vi "1. Basic retrieve Rulers.vi"() -> ()   [LabVIEW 2017]
uses:
  40fc1cc9-77e3-4a14-9bb9-de70462c7f35.vi
  81b41104-5ca5-45e9-a143-87b761583821.vi
  83982d16-e29d-493a-892c-93b6b063dd3a.vi
  d59d594f-6358-4fe9-a0ea-ade5f599e91a.vi
  177f037c-d6c1-4684-97ba-f775e359171c.vi
  f8914412-5770-4d7c-8ed9-34d3b6c64140.vi
  0842be61-58c2-4c06-9355-20aaf40be817.vi
  a49a9376-e1ff-4fda-bff8-7fdb6b491f6f.vi
  efc68658-e21b-4998-9bfe-a9de0054dd82.vi
  38ed8c4c-bfe5-4ceb-af5c-8de10cee5e52.vi
  a345cc07-d10f-4275-8a18-17707c3f89e9.vi
  cabc4c38-4671-4b03-9489-31c074b0dc0c.vi
  API-String-Arugments-Support/_Support/Convert API String Arguments to Data(variant).vi
panel:
  out "output cluster 11":T1={"API String"="[3.12,4.113,2.3,5;3.12,5,2.3;3.12,4.11,5]", "2D DBL"=[[3.12, 4.113, 2.3, 5.0, 5.0, 2.3, 4.11, 5.0]], "Retrieved Data"=[[3.12, 4.113, 2.3, 5.0], [3.12, 5.0, 2.3, 0.0], [3.12, 4.11, 5.0, 0.0]]}
  out "output cluster 10":T2={"API String"="[{Bool:Off;child.name:ddd},{Bool:On;name:ddd}]", "Cluster Array"=[{"Name"="x", "Child"={"Name"="xxx"}, "Bool"=TRUE}, {"Name"="xxx", "Child"={"Name"="x"}, "Bool"=FALSE}], "Retrieved Data"=[{"Name"="", "Child"={"Name"="ddd"}, "Bool"=FALSE}, {"Name"="ddd", "Child"={"Name"=""}, "Bool"=TRUE}]}
  out "output cluster 9":T3={"API String"="Bool:Off;child.name:ddd", "Cluster"={"Name"="abc", "Child"={"Name"="xxx"}, "Bool"=TRUE}, "Retrieved Data"={"Name"="abc", "Child"={"Name"="ddd"}, "Bool"=FALSE}}
  out "output cluster 8":T4={"API String"="[3.12,4.11,5]", "1D DBL"=[0.0, 0.0, 0.0], "Retrieved Data"=[3.12, 4.11, 5.0]}
  out "output cluster 7":T5={"API String"="555", "Enum"=enum."1 - aaaa", "Retrieved Data"=enum."555 - ccccc"}
  out "output cluster 6":T5={"API String"="bbbb", "Enum"=enum."1 - aaaa", "Retrieved Data"=enum."2 - bbbb"}
  out "output cluster 5":T6={"API String"="bbbb", "Enum"=enum."aaaa", "Retrieved Data"=enum."bbbb"}
  out "output cluster 4":T7={"API String"="3.1415926", "DBL"=3.1415926, "Retrieved Data"=3.1415926}
  out "output cluster 3":T8={"API String"="0x42", "I32"=0, "Retrieved Data"=66}
  out "output cluster 2":T9={"API String"="Enable", "Boolean"=FALSE, "Retrieved Data"=TRUE}
  out "output cluster":T10={"API String"="abcd", "String"="", "Retrieved Data"="abcd"}
  out "output":T11={"API String"="C:\\ni-rt\\data\\a\\2025.08.25", "Path"=path "C:/ni-rt/a", "Retrieved Data"=path "C:/ni-rt/data/a/2025.08.25"}
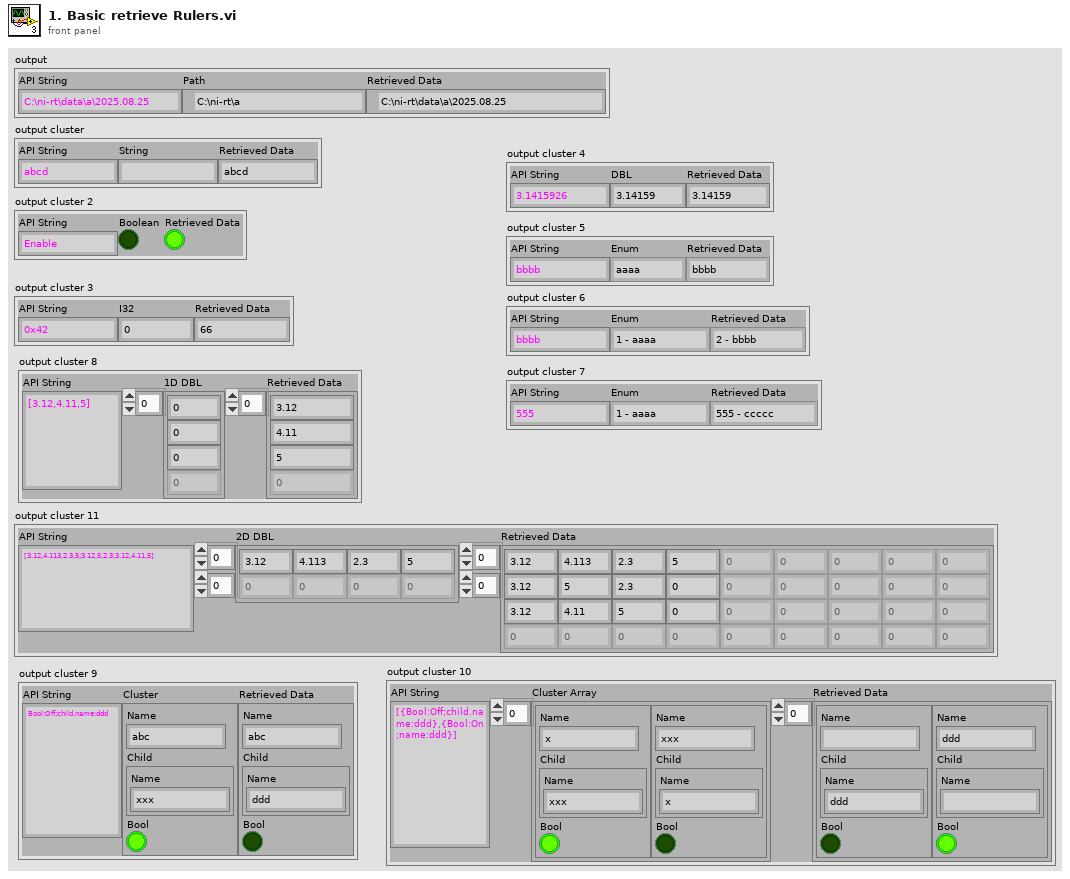
[diagram p1: front panel]
types:
  T1 = cluster{"API String":string, "2D DBL":dbl[][], "Retrieved Data":dbl[][]}
  T2 = cluster{"API String":string, "Cluster Array":cluster{"Name":string, "Child":cluster{"Name":string}, "Bool":bool}[], "Retrieved Data":cluster{"Name":string, "Child":cluster{"Name":string}, "Bool":bool}[]}
  T3 = cluster{"API String":string, "Cluster":cluster{"Name":string, "Child":cluster{"Name":string}, "Bool":bool}, "Retrieved Data":cluster{"Name":string, "Child":cluster{"Name":string}, "Bool":bool}}
  T4 = cluster{"API String":string, "1D DBL":dbl[], "Retrieved Data":dbl[]}
  T5 = cluster{"API String":string, "Enum":enum16{"1 - aaaa", "2 - bbbb", "555 - ccccc"}, "Retrieved Data":enum16{"1 - aaaa", "2 - bbbb", "555 - ccccc"}}
  T6 = cluster{"API String":string, "Enum":enum16{"aaaa", "bbbb", "ccccc"}, "Retrieved Data":enum16{"aaaa", "bbbb", "ccccc"}}
  T7 = cluster{"API String":string, "DBL":dbl, "Retrieved Data":dbl}
  T8 = cluster{"API String":string, "I32":i32, "Retrieved Data":i32}
  T9 = cluster{"API String":string, "Boolean":bool, "Retrieved Data":bool}
  T10 = cluster{"API String":string, "String":string, "Retrieved Data":string}
  T11 = cluster{"API String":string, "Path":path, "Retrieved Data":path}
  T12 = cluster{"Name":string, "Child":cluster{"Name":string}, "Bool":bool}[]
  T13 = cluster{"Name":string, "Child":cluster{"Name":string}, "Bool":bool}
  T14 = cluster{"String":string, "Data 9":path, "Data":path}
  T15 = cluster{"String":string, "Data 1":string, "Data":string}
  T16 = cluster{"String":string, "Data 2":bool, "Data":bool}
  T17 = cluster{"String":string, "Data 3":i32, "Data":i32}
  T18 = cluster{"String":string, "Data 4":dbl, "Data":dbl}
  T19 = cluster{"String":string, "Data 5":enum16{"aaaa", "bbbb", "ccccc"}, "Data":enum16{"aaaa", "bbbb", "ccccc"}}
  T20 = cluster{"String":string, "Data 6":enum16{"1 - aaaa", "2 - bbbb", "555 - ccccc"}, "Data":enum16{"1 - aaaa", "2 - bbbb", "555 - ccccc"}}
  T21 = cluster{"String":string, "Data 7":enum16{"1 - aaaa", "2 - bbbb", "555 - ccccc"}, "Data":enum16{"1 - aaaa", "2 - bbbb", "555 - ccccc"}}
  T22 = cluster{"String":string, "Data 4":dbl[], "Data":dbl[]}
  T23 = cluster{"String":string, "Data 8":cluster{"Name":string, "Child":cluster{"Name":string}, "Bool":bool}, "Data":cluster{"Name":string, "Child":cluster{"Name":string}, "Bool":bool}}
  T24 = cluster{"String":string, "Data 10":cluster{"Name":string, "Child":cluster{"Name":string}, "Bool":bool}[], "Data":cluster{"Name":string, "Child":cluster{"Name":string}, "Bool":bool}[]}
  T25 = cluster{"String":string, "Data 11":dbl[][], "Data":dbl[][]}
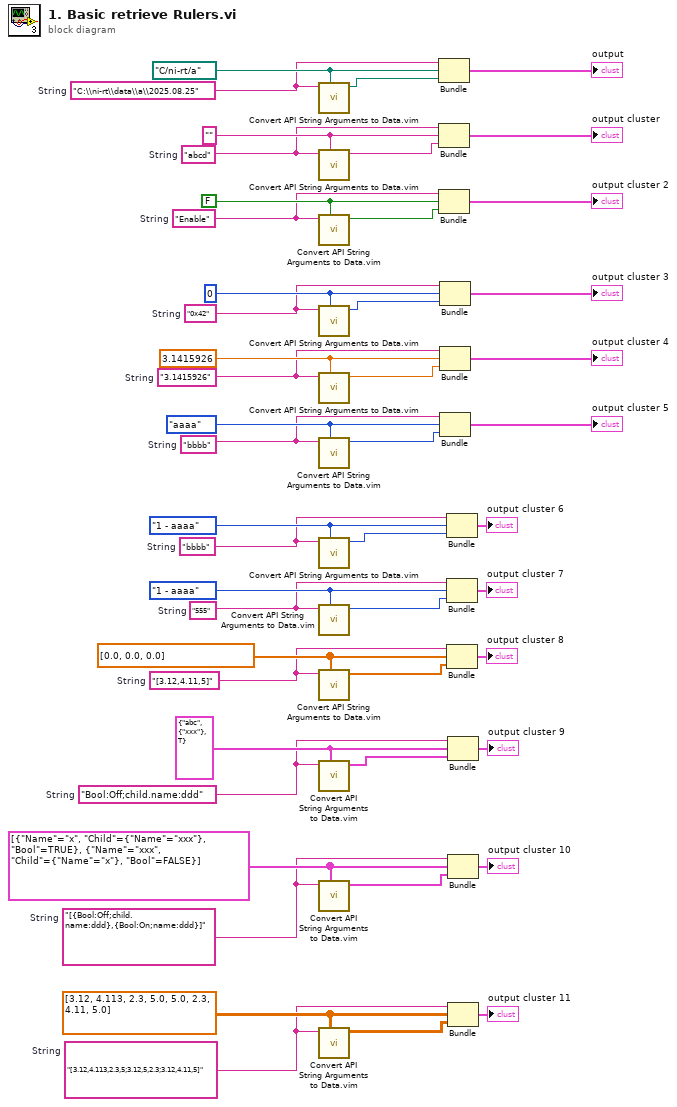
[diagram p0: block diagram]
diagram:
  w1 = "[3.12,4.113,2.3,5;3.12,5,2.3;3.12,4.11,5]"  # String
  w2 = "[{Bool:Off;child.name:ddd},{Bool:On;name:ddd}]"  # String
  w3 = "Bool:Off;child.name:ddd"  # String
  w4 = "[3.12,4.11,5]"  # String
  w5 = "555"  # String
  w6 = "bbbb"  # String
  w7 = "bbbb"  # String
  w8 = "3.1415926"  # String
  w9 = "0x42"  # String
  w10 = "Enable"  # String
  w11 = "abcd"  # String
  w18 = dbl[][] [[3.12, 4.113, 2.3, 5.0, 5.0, 2.3, 4.11, 5.0]] ("Data 11")
  w19 = T12 [{"Name"="x", "Child"={"Name"="xxx"}, "Bool"=TRUE}, {"Name"="xxx", "Child"={"Name"="x"}, "Bool"=FALSE}] ("Data 10")
  w20 = T13 {"Name"="abc", "Child"={"Name"="xxx"}, "Bool"=TRUE} ("Data 8")
  w21 = dbl[] [0.0, 0.0, 0.0] ("Data 4")
  w22 = enum16{"1 - aaaa", "2 - bbbb", "555 - ccccc"}."1 - aaaa" ("Data 7")
  w23 = enum16{"1 - aaaa", "2 - bbbb", "555 - ccccc"}."1 - aaaa" ("Data 6")
  w34 = enum16{"aaaa", "bbbb", "ccccc"}."aaaa" ("Data 5")
  w35 = 3.1415926 ("Data 4")
  w36 = 0 ("Data 3")
  w41 = FALSE ("Data 2")
  w45 = "" ("Data 1")
  w48 = path "C:/ni-rt/a" ("Data 9")
  w24 = "C:\\ni-rt\\data\\a\\2025.08.25"  # String
  n1 = call "Convert API String Arguments to Data.vim"("Type"=w48, "String"=w24) -> ("Data"=w47:path)  [unwired: 6 in, 1 out]
  n2 = call "Convert API String Arguments to Data.vim"("Type"=w45, "String"=w11) -> ("Data"=w44:string)  [unwired: 6 in, 1 out]
  n3 = call "Convert API String Arguments to Data.vim"("Type"=w41, "String"=w10) -> ("Data"=w42:bool)  [unwired: 6 in, 1 out]
  n4 = call "Convert API String Arguments to Data.vim"("Type"=w36, "String"=w9) -> ("Data"=w37:i32)  [unwired: 6 in, 1 out]
  n5 = call "Convert API String Arguments to Data.vim"("Type"=w35, "String"=w8) -> ("Data"=w38:dbl)  [unwired: 6 in, 1 out]
  n6 = call "Convert API String Arguments to Data.vim"("Type"=w34, "String"=w7) -> ("Data"=w39:enum16{"aaaa", "bbbb", "ccccc"})  [unwired: 6 in, 1 out]
  n7 = call "Convert API String Arguments to Data.vim"("Type"=w23, "String"=w6) -> ("Data"=w25:enum16{"1 - aaaa", "2 - bbbb", "555 - ccccc"})  [unwired: 6 in, 1 out]
  n8 = call "Convert API String Arguments to Data.vim"("Type"=w22, "String"=w5) -> ("Data"=w26:enum16{"1 - aaaa", "2 - bbbb", "555 - ccccc"})  [unwired: 6 in, 1 out]
  n9 = call "Convert API String Arguments to Data.vim"("Type"=w21, "String"=w4) -> ("Data"=w27:dbl[])  [unwired: 6 in, 1 out]
  n10 = call "Convert API String Arguments to Data.vim"("Type"=w20, "String"=w3) -> ("Data"=w30:T13)  [unwired: 6 in, 1 out]
  n11 = call "Convert API String Arguments to Data.vim"("Type"=w19, "String"=w2) -> ("Data"=w29:T12)  [unwired: 6 in, 1 out]
  n12 = call "Convert API String Arguments to Data.vim"("Type"=w18, "String"=w1) -> ("Data"=w28:dbl[][])  [unwired: 6 in, 1 out]
  n13 = Bundle("String"=w24, "Data 9"=w48, "Data"=w47) -> (→"output":T14)  [unwired: 1 in]
  n14 = Bundle("String"=w11, "Data 1"=w45, "Data"=w44) -> (→"output cluster":T15)  [unwired: 1 in]
  n15 = Bundle("String"=w10, "Data 2"=w41, "Data"=w42) -> (→"output cluster 2":T16)  [unwired: 1 in]
  n16 = Bundle("String"=w9, "Data 3"=w36, "Data"=w37) -> (→"output cluster 3":T17)  [unwired: 1 in]
  n17 = Bundle("String"=w8, "Data 4"=w35, "Data"=w38) -> (→"output cluster 4":T18)  [unwired: 1 in]
  n18 = Bundle("String"=w7, "Data 5"=w34, "Data"=w39) -> (→"output cluster 5":T19)  [unwired: 1 in]
  n19 = Bundle("String"=w6, "Data 6"=w23, "Data"=w25) -> (→"output cluster 6":T20)  [unwired: 1 in]
  n20 = Bundle("String"=w5, "Data 7"=w22, "Data"=w26) -> (→"output cluster 7":T21)  [unwired: 1 in]
  n21 = Bundle("String"=w4, "Data 4"=w21, "Data"=w27) -> (→"output cluster 8":T22)  [unwired: 1 in]
  n22 = Bundle("String"=w3, "Data 8"=w20, "Data"=w30) -> (→"output cluster 9":T23)  [unwired: 1 in]
  n23 = Bundle("String"=w2, "Data 10"=w19, "Data"=w29) -> (→"output cluster 10":T24)  [unwired: 1 in]
  n24 = Bundle("String"=w1, "Data 11"=w18, "Data"=w28) -> (→"output cluster 11":T25)  [unwired: 1 in]
